vi "Launch Top Level Modules.vi"(8 "error in (no error)":errorcluster, 11 "Volatus Core in":refnum<class "Volatus Core.lvclass">) -> (0 "error out":errorcluster, 3 "Volatus Core out":refnum<class "Volatus Core.lvclass">)   [LabVIEW 2020, in "Volatus.lvlib" / "Volatus Core.lvclass"]
uses:
  Volatus Core.lvclass
  C:/dev/lv20CE/relink/lv-volatus/Volatus/Module/Module.lvclass
  Module/Module.lvclass/Module.ctl
  VolatusConfig/VolatusConfigElement/VolatusConfigElement.lvclass/VolatusConfigElement.ctl
  VolatusConfig/VolatusConfigElement/Element.vi
  lv-cdm/CDM-Config/Config Element/Lookup Child by Name.vi
  Volatus Core.lvclass/Volatus Core.ctl
  VolatusAPI/VolatusAPI.lvclass
  Module/Module.lvclass
  VolatusConfig/Node/Node.lvclass
  VolatusConfig/Task/Task.lvclass
  C:/dev/lv20CE/relink/lv-volatus/VolatusConfig/VolatusConfigElement/VolatusConfigElement.lvclass
  C:/dev/lv20CE/relink/lv-volatus/VolatusConfig/Task/Task.lvclass
  C:/dev/lv20CE/relink/lv-volatus/Volatus/Volatus Core/Volatus Core.lvclass
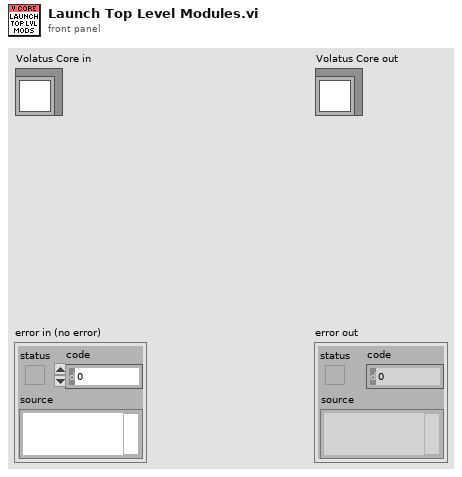
[diagram p1: front panel]
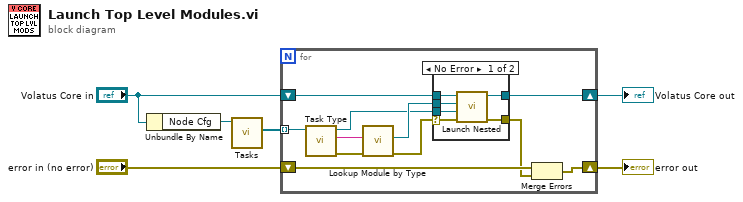
[diagram p0: block diagram]
diagram:
  n1 = Unbundle By Name("Volatus Core in") -> ("Node Cfg"=w4:refnum<class "Node.lvclass">)
  n2 = call "Tasks.vi"("Node in"=w4) -> ("Tasks"=w3:refnum<class "Task.lvclass">[])  [unwired: 8 in, 2 out]
  n3 = for {
    tunnel: w3 -> [w10] mode=indexing
    shift-right: [w14] -> w5
    shift-left: "Volatus Core in" -> [w17]
    shift-right: [w11] -> w6
    shift-left: "error in (no error)" -> [w13]
    n4 = call "Task Type.vi"("Task in"=w10) -> ("error out"=w7:errorcluster, "Task Type"=w8:string, "Task out"=w9:refnum<class "Task.lvclass">)  [unwired: 8 in]
    n5 = call "Lookup Module by Type.vi"("error in (no error)"=w7, "Module Type"=w8) -> ("error out"=w15:errorcluster, "Module"=w16:refnum<class "Module.lvclass">)  [unwired: 8 in]
    n6 = case shown="No Error" w15 {
      selector: w15 -> [w20 w24]
      tunnel: w17 -> [w23 w25]
      tunnel: w16 -> [w22 _]
      tunnel: w9 -> [w21 _]
      tunnel: [w19 w24] -> w12
      tunnel: [w18 w25] -> w14
      frame No Error {
        n7 = call "Launch Nested.vi"("error in (no error)"=w20, "Config Element"=w21, "Nested Module"=w22, "Parent in"=w23) -> ("error out"=w19:errorcluster, "Parent out"=w18:refnum<class "Volatus Core.lvclass">)  [unwired: 5 in, 1 out]
      }
      frame Error {
      }
    }
    n8 = Merge Errors(w13, w12) -> (w11:errorcluster)
  }
  "error out" <- w6
  "Volatus Core out" <- w5
